vi "Check All Value Changed.vi"(8 "error in (no error)":errorcluster, 10 "New Value":bool, 11 "MCListbox with Checkboxes in":refnum<class "MCListbox with Checkboxes.lvclass">) -> (0 "error out":errorcluster, 3 "MCListbox with Checkboxes out":refnum<class "MCListbox with Checkboxes.lvclass">)   [LabVIEW 2016, in "MCListbox with Checkboxes.lvclass"]
uses:
  MCListbox with Checkboxes.lvclass
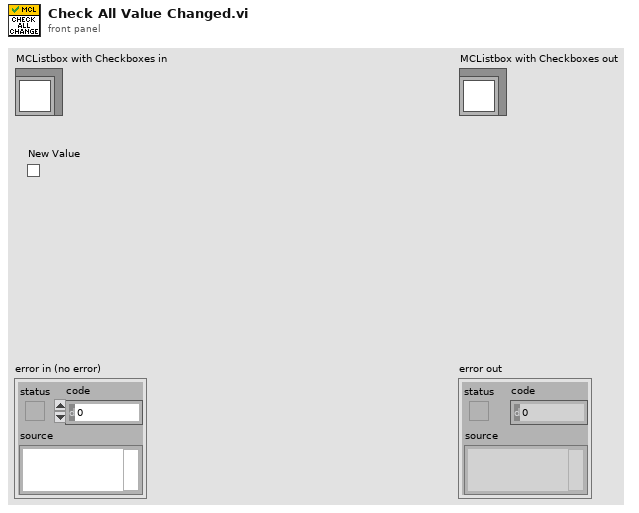
[diagram p1: front panel]
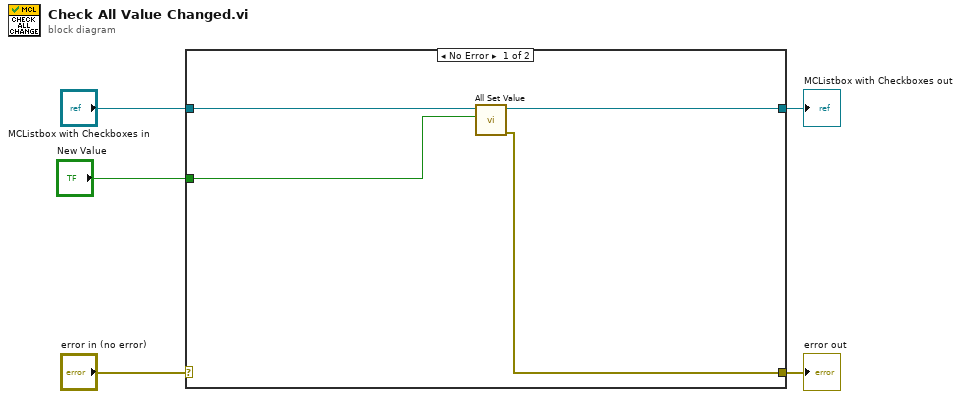
[diagram p0: block diagram]
diagram:
  n1 = case shown="No Error" "error in (no error)" {
    selector: "error in (no error)" -> [_ w11]
    tunnel: [w7 w11] -> w4
    tunnel: [w8 w10] -> w2
    tunnel: "MCListbox with Checkboxes in" -> [w9 w10]
    tunnel: "New Value" -> [w6 _]
    frame No Error {
      n2 = call "All Set Value.vi"("Value (F)"=w6, "MCListbox with Checkboxes in"=w9) -> ("error out"=w7:errorcluster, "MCListbox with Checkboxes out"=w8:refnum<class "MCListbox with Checkboxes.lvclass">)  [unwired: 8 in]
    }
    frame Error {
    }
  }
  "error out" <- w4
  "MCListbox with Checkboxes out" <- w2
